vi "Do.vi"(8 "error in (no error)":errorcluster, 10 "Actor in":refnum<class "Actor.lvclass">, 11 "Quench Msg":refnum<class "Quench Msg.lvclass">) -> (0 "error out":errorcluster, 2 "Actor out":refnum<class "Actor.lvclass">)   [LabVIEW 2016, in "KIT-QVA.lvlib" / "Quench Msg.lvclass"]
doc: "This VI delivers the message to the actor by calling the appropriate method(s) on the actor."
uses:
  Quench Msg.lvclass
  <vilib>/ActorFramework/Actor/Actor.lvclass
  C:/User/Brand/LVP/STF/Packages/CSPP_Core/Actors/CS++PVMonitor Messages/CS++PVUpdate Msg/CS++PVUpdate Msg.lvclass
  KIT-QVA/KIT-QVA.lvclass
  C:/Program Files (x86)/National Instruments/LabVIEW 2016/vi.lib/ActorFramework/Actor/Actor.lvclass
  CSPP_Core/Actors/CS++PVMonitor Messages/CS++PVUpdate Msg/CS++PVUpdate Msg.lvclass/CS++PVUpdate Msg.ctl
  CSPP_Core/Classes/CS++ProcessVariables/ProcessVariable/PV.lvclass/PV.ctl
  Quench Msg.lvclass/Quench Msg.ctl
  CSPP_Core/Classes/CS++ProcessVariables/ProcessVariable/PV.lvclass
  CSPP_Core/Actors/CS++PVMonitor Messages/CS++PVUpdate Msg/CS++PVUpdate Msg.lvclass
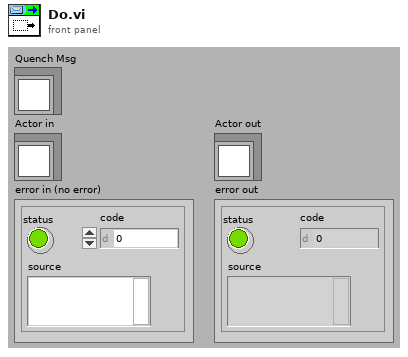
[diagram p1: front panel]
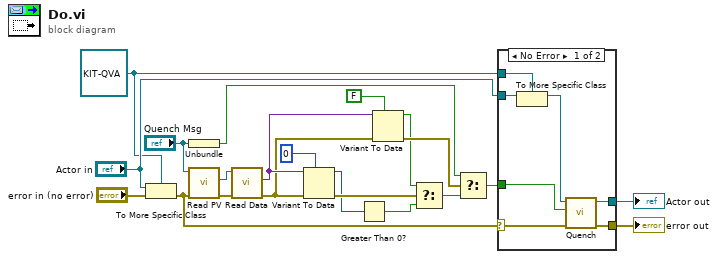
[diagram p0: block diagram]
diagram:
  w17 = refnum<class "KIT-QVA.lvclass"> refnum ("Actor in")
  n1 = To More Specific Class(target class=w17, reference="Actor in", error in="error in (no error)") -> (error out=w5:errorcluster)  [unwired: 1 out]
  n2 = Unbundle ("Pre-Unbundler")("Quench Msg") -> (w1:bool)
  n3 = call "Read PV.vi"("error in (no error)"=w5, "CS++PVUpdate Msg in"="Quench Msg") -> ("error out"=w16:errorcluster, "PV"=w13:refnum<class "PV.lvclass">)  [unwired: 7 in, 1 out]
  n4 = call "Read Data.vi"("error in (no error)"=w16, "PV in"=w13) -> ("error out"=w10:errorcluster, "Data"=w11:variant)  [unwired: 7 in, 1 out]
  n5 = Variant To Data ("I16-Conversion")(error in=w10, type=i16 0 ("I16-Conversion-Constant"), Variant=w11) -> (data=w4:i16, error out=w9:errorcluster)
  n6 = Greater Than 0? ("I16-Comp0")(x=w4) -> (x > 0?=w3:bool)
  n7 = Variant To Data(error in=w10, type=FALSE ("Quench"), Variant=w11) -> (data=w8:bool, error out=w15:errorcluster)
  n8 = Select ("I16-Select")(t=w8, s=w9, f=w3) -> (s? t:f=w7:bool)
  n9 = Select ("MainSelect")(t=w1, s=w15, f=w7) -> (s? t:f=w2:bool)
  n10 = case shown="No Error" w5 {
    selector: w5 -> [w26 w30]
    tunnel: [w28 w30] -> w20
    tunnel: [w27 w29] -> w19
    tunnel: "Actor in" -> [w25 w29]
    tunnel: w17 -> [w24 _]
    tunnel: w2 -> [w22 _]
    frame No Error {
      n11 = To More Specific Class(target class=w24, reference=w25) -> (specific class reference=w23:refnum<class "KIT-QVA.lvclass">)  [unwired: 1 in, 1 out]
      n12 = call "Quench.vi"("Error In"=w26, "Quench"=w22, "KIT-QVA in"=w23) -> ("Error Out"=w28:errorcluster, "KIT-QVA out"=w27:refnum<class "KIT-QVA.lvclass">)  [unwired: 7 in]
    }
    frame Error {
    }
  }
  "error out" <- w20
  "Actor out" <- w19
